vi "수업3.vi"() -> ()   [LabVIEW 2014]
panel:
  out "배열":dbl[](array[numeric])
  in  "숫자형 2":dbl
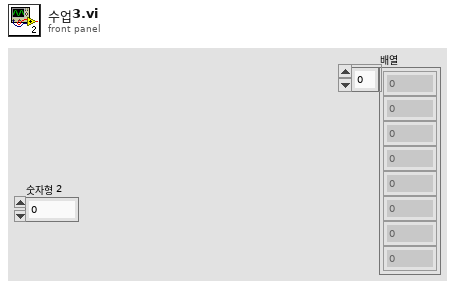
[diagram p1: front panel]
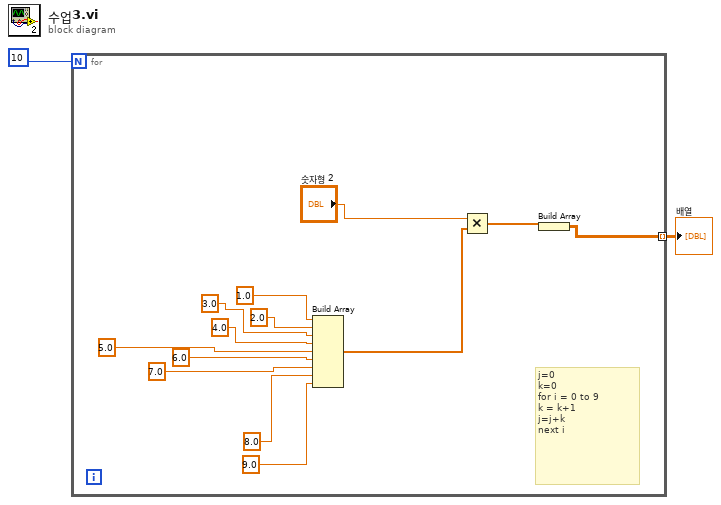
[diagram p0: block diagram]
diagram:
  n1 = for {
    N: 10 -> [_]
    tunnel: [w15] -> w1 mode=indexing
    # "j=0\nk=0\nfor i = 0 to 9\nk = k+1\nj=j+k\nnext i"
    n2 = Build Array(1.0 ("y"), 2.0 ("y"), 3.0 ("y"), 4.0 ("y"), 5.0 ("y"), 6.0 ("y"), 7.0 ("y"), 8.0 ("y"), 9.0 ("y")) -> (w4:dbl[])
    n3 = Multiply(x="숫자형 2", y=w4) -> (x*y=w14:dbl[])
    n4 = Build Array(w14) -> (w15:dbl[][])
  }
  "배열" <- w1
